vi "T_Sat_Curve_Fit_R245fa.vi"(11 "Dynamic Data in":dynamicdata(waveform)) -> (3 "Dynamic Data out":dynamicdata(waveform))   [LabVIEW 2016]
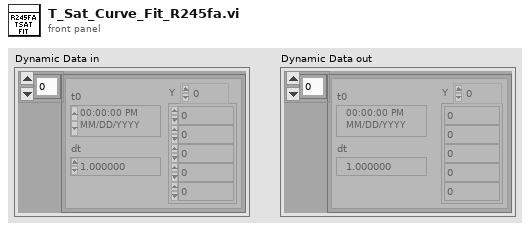
[diagram p1: front panel]
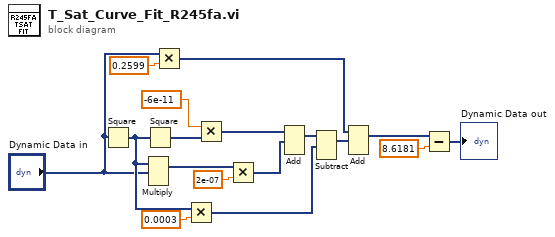
[diagram p0: block diagram]
diagram:
  n1 = Square(x="Dynamic Data in") -> (x^2=w11:dynamicdata)
  n2 = Multiply(1:"Dynamic Data in", 2:w11) -> (0:w16:dynamicdata)  [unwired: 1 in, 1 out]
  n3 = Square(x=w11) -> (x^2=w13:dynamicdata)
  n4 = Multiply(x="Dynamic Data in", y=0.2599) -> (x*y=w5:dynamicdata)
  n5 = Multiply(x=w11, y=0.0003) -> (x*y=w9:dynamicdata)
  n6 = Multiply(x=-6e-11 ("y"), y=w13) -> (x*y=w12:dynamicdata)
  n7 = Multiply(x=w16, y=2e-07) -> (x*y=w14:dynamicdata)
  n8 = Add(1:w14, 2:w12) -> (0:w8:dynamicdata)  [unwired: 1 in, 1 out]
  n9 = Subtract(1:w9, 2:w8) -> (0:w4:dynamicdata)  [unwired: 1 in, 1 out]
  n10 = Add(1:w4, 2:w5) -> (0:w2:dynamicdata)  [unwired: 1 in, 1 out]
  n11 = Subtract(x=w2, y=8.6181) -> (x-y=→"Dynamic Data out":dynamicdata)
